vi "快捷购买.vi"() -> ()   [LabVIEW 2020]
panel:
  out "地址： 2":string
  out "电话： 2":string
  in  "确认":bool
  in  "地址：":string
  in  "电话：":string
  # "请填写以下信息"
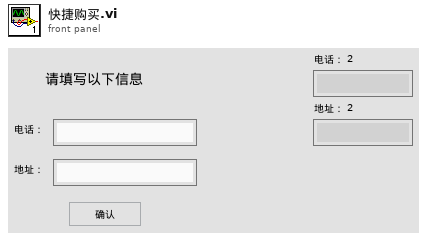
[diagram p1: front panel]
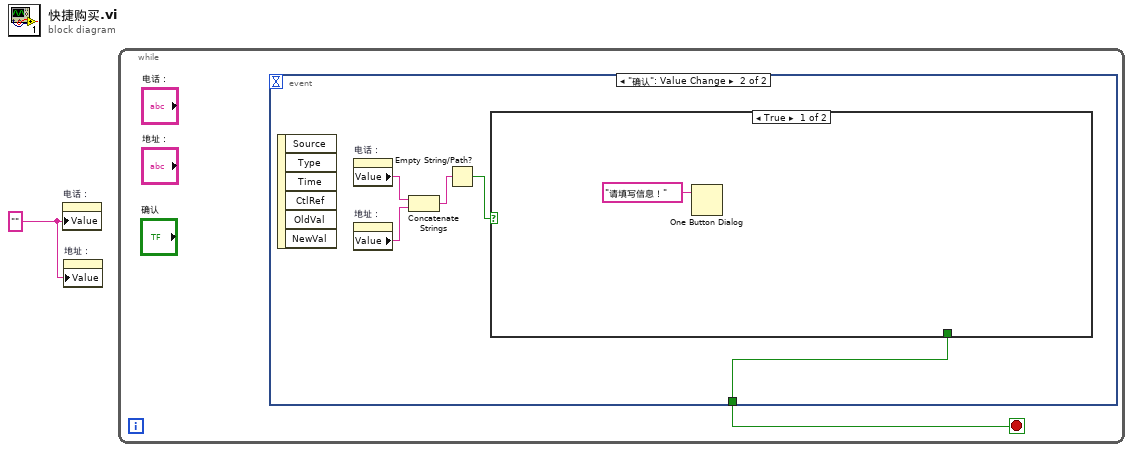
[diagram p0: block diagram]
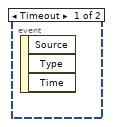
[diagram p2: hidden frame]
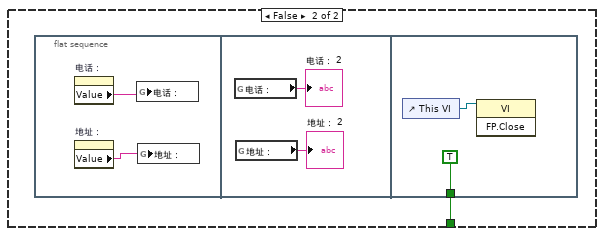
[diagram p3: hidden frame]
diagram:
  w1 = "" ("电话：")
  n1 = property on="电话：" class="Str"("Value"=w1) -> ()  [unwired: 2 in, 2 out]
  n2 = property on="地址：" class="Str"("Value"=w1) -> ()  [unwired: 2 in, 2 out]
  n3 = while {
    stop <- w2 stop-if-true
    n4 = event shown="[1] \"确认\": Value Change" {
      selector: _ -> [_ _]
      dyn-events: _ -> [_ _]
      timeout: _ -> [_ _]
      tunnel: [_ w7] -> w2
      event Timeout {
        n5 = event-data() -> ()  [unwired: 1 in, 3 out]
      }
      event "确认": Value Change {
        n6 = event-data() -> ()  [unwired: 1 in, 6 out]
        n7 = property on="电话：" class="Str"() -> ("Value"=w5:string)  [unwired: 2 in, 2 out]
        n8 = property on="地址：" class="Str"() -> ("Value"=w4:string)  [unwired: 2 in, 2 out]
        n9 = Concatenate Strings(w5, w4) -> (w6:string)
        n10 = Empty String/Path?(string/path=w6) -> (empty?=w3:bool)
        n11 = case shown="True" w3 {
          tunnel: [_ w9] -> w7
          frame True {
            n12 = One Button Dialog(message="请填写信息！") -> ()  [unwired: 1 in, 1 out]
          }
          frame False {
            n13 = flat-sequence {
              tunnel: [TRUE] -> w9
              frame #0 {
                n14 = property on="电话：" class="Str"() -> ("Value"=w11:string)  [unwired: 2 in, 2 out]
                n15 = property on="地址：" class="Str"() -> ("Value"=w10:string)  [unwired: 2 in, 2 out]
                n16 = global write "快捷购买信息.vi" "电话："(w11) -> ()
                n17 = global write "快捷购买信息.vi" "地址："(w10) -> ()
              }
              frame #1 {
                n18 = global read "快捷购买信息.vi" "电话："() -> (→"电话： 2":string)
                n19 = global read "快捷购买信息.vi" "地址："() -> (→"地址： 2":string)
              }
              frame #2 {
                n20 = control-ref of="This VI"() -> (w14:refnum<vi>)
                n21 = invoke class="VI" method="FP.Close"(reference=w14) -> ()  [unwired: 2 in, 3 out]
              }
            }
          }
        }
      }
    }
  }
